vi "Write Header.vi"(8 "error in (no error)":errorcluster, 10 "Header":T1, 11 "TCPPacket in":refnum<class "TCPPacket.lvclass">) -> (0 "error out":errorcluster, 3 "TCPPacket out":refnum<class "TCPPacket.lvclass">)   [LabVIEW 2019, in "TCPPacket.lvclass"]
uses:
  TCPPacket.lvclass
  TCPHeader STYP.ctl
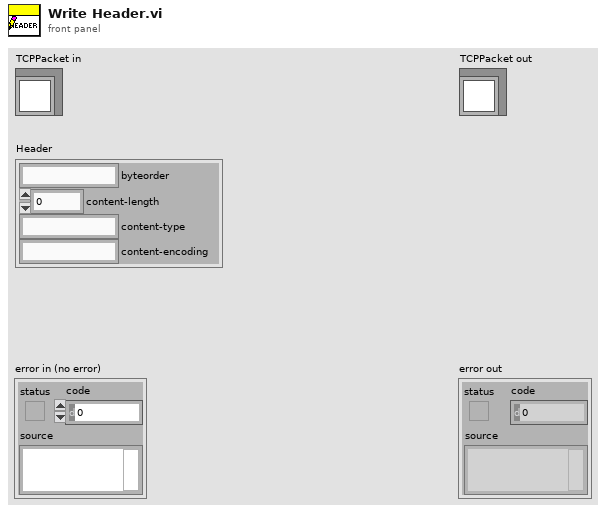
[diagram p1: front panel]
types:
  T1 = typedef "TCPPacket.lvclass/TCPHeader STYP.ctl" = cluster{"byteorder":string, "content-length":u32, "content-type":string, "content-encoding":string}
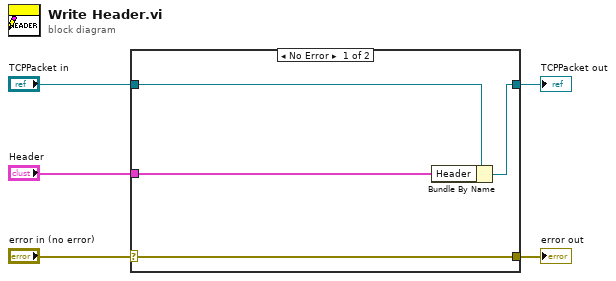
[diagram p0: block diagram]
diagram:
  n1 = case shown="No Error" "error in (no error)" {
    selector: "error in (no error)" -> [w9 w10]
    tunnel: [w9 w10] -> w4
    tunnel: [w7 w11] -> w2
    tunnel: "TCPPacket in" -> [w8 w11]
    tunnel: "Header" -> [w6 _]
    frame No Error {
      n2 = Bundle By Name(cluster=w8, "Header"=w6) -> (w7:refnum<class "TCPPacket.lvclass">)
    }
    frame Error {
    }
  }
  "error out" <- w4
  "TCPPacket out" <- w2
